vi "20170411-lecture3-multi read write local variable problem.vi"() -> ()   [LabVIEW 2014]
panel:
  in  "x":dbl
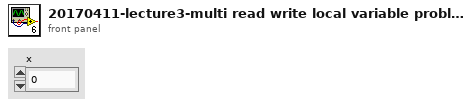
[diagram p1: front panel]
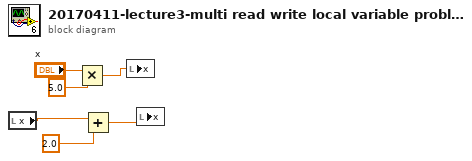
[diagram p0: block diagram]
diagram:
  n1 = local read "x"() -> (w1:dbl)
  n2 = Multiply(x="x", y=5.0) -> (x*y=w3:dbl)
  n3 = Add(x=w1, y=2.0) -> (x+y=w2:dbl)
  n4 = local write "x"(w3) -> ()
  n5 = local write "x"(w2) -> ()
